vi "to string.vi"(8 "error in":errorcluster, 11 "configuration in":refnum<class "action configuration.lvclass">) -> (0 "error out":errorcluster, 1 "data":string, 2 "version":string, 3 "configuration out":refnum<class "action configuration.lvclass">)   [LabVIEW 2015, in "action configuration.lvclass"]
doc: "Provides an interface for saving a module configuration to a file or other serialized data source. It is recommended that all children of this class store data in two sets--data required for its own initialization, and any data required for parent initialization--and that each implementation uses the <b>Call Parent Method</b> primitive to serialize parent information."
uses:
  action configuration.lvclass
  <vilib>/NI/Tag Bus Module Framework/root configuration/TBM configuration.lvclass
  <vilib>/NI/Configuration Framework/serializable configuration/NISE_CEF_serializable configuration.lvclass
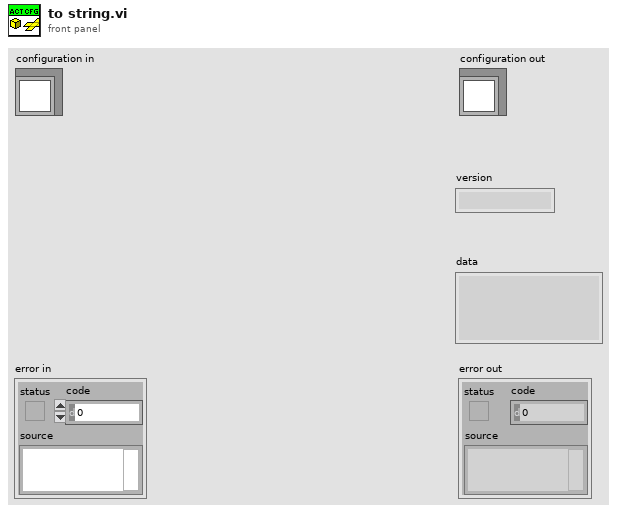
[diagram p1: front panel]
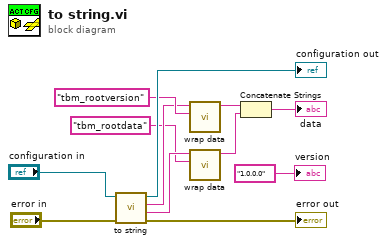
[diagram p0: block diagram]
diagram:
  n1 = call-parent "to string.vi"("error in"="error in", "configuration in"="configuration in") -> ("error out"=→"error out":errorcluster, "data"=w2:string, "version"=w4:string, "configuration out"=→"configuration out":refnum<class "action configuration.lvclass">)  [unwired: 6 in]
  n2 = call <vilib>:"wrap data.vi"("identifier"="tbm_rootversion" ("additional identifier"), "data to wrap"=w4) -> ("wrapped data"=w6:string)  [unwired: 9 in]
  n3 = call <vilib>:"wrap data.vi"("identifier"="tbm_rootdata" ("additional identifier"), "data to wrap"=w2) -> ("wrapped data"=w3:string)  [unwired: 9 in]
  n4 = Concatenate Strings(w6, w3) -> (→"data":string)
  "version" <- "1.0.0.0" ("version")
